vi "写内部参数解析.vi"(9 "读取的字节":i32, 10 "响应":string) -> (2 "内部参数":string[](array[string]))   [LabVIEW 2020]
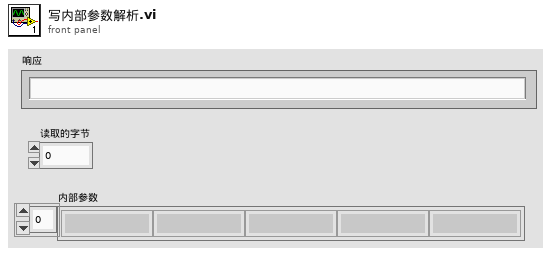
[diagram p1: front panel]
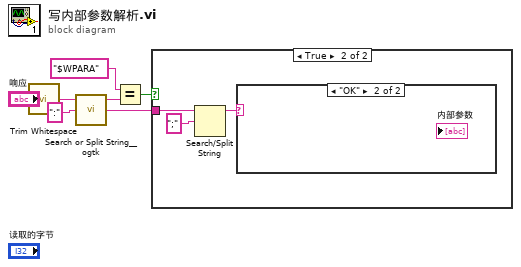
[diagram p0: block diagram]
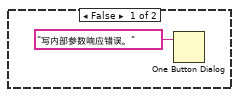
[diagram p2: hidden frame]
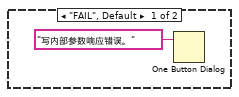
[diagram p3: hidden frame]
diagram:
  n1 = call <vilib>:"Trim Whitespace.vi"("string"="响应") -> ("trimmed string"=w1:string)  [unwired: 1 in]
  n2 = call <userlib>:"Search or Split String__ogtk.vi"("search string/char (-)"=":", "string"=w1) -> ("substring after match"=w2:string, "substring before match"=w5:string)  [unwired: 1 in, 1 out]
  n3 = Equal?(x="$WPARA" ("search string/char (-)"), y=w5) -> (x = y?=w3:bool)
  n4 = case shown="True" w3 {
    tunnel: w2 -> [_ w10]
    frame False {
      n5 = One Button Dialog(message="写内部参数响应错误。" ("消息")) -> ()  [unwired: 1 in, 1 out]
    }
    frame True {
      n6 = Search/Split String(string=w10, search string/char (-)=";" ("搜索字符串/字符(-)")) -> (substring before match=w9:string)  [unwired: 1 in, 2 out]
      n7 = case shown="\"OK\"" w9 {
        frame "FAIL", Default {
          n8 = One Button Dialog(message="写内部参数响应错误。" ("消息")) -> ()  [unwired: 1 in, 1 out]
        }
        frame "OK" {
        }
      }
    }
  }
